vi "Velocity Profile.vi"(0 "Set Point":dbl(slide)=1510.204081632653 scale=-2000.0..2000.0, 1 "Iteration":i32, 2 "Reset":bool, 3 "Reset 2":bool, 5 "Position Sense":dbl(slide) scale=-2000.0..2000.0, 7 "Rate Sense":dbl(slide) scale=-1000.0..1000.0, 11 "Velocity Profile":dbl[][](array[numeric])=[[50.0, 75.0, 0.05], [100.0, 150.0, 0.1], [250.0, 400.0, 0.2], [500.0, inf, 0.2]], 12 "queue":refnum<queue>, 13 "Hold":bool, 14 "array":dbl[](array[numeric])) -> (4 "Motor":dbl, 8 "arrived":bool, 15 "gear":i32)   [LabVIEW 2012]
panel:
  out "Rate Obj":dbl(graph)
  out "Accel":dbl
  out "Rate":dbl
  out "Waveform Chart":dbl(graph)
  # "Range"
  # "Rate"
  # "Accel"
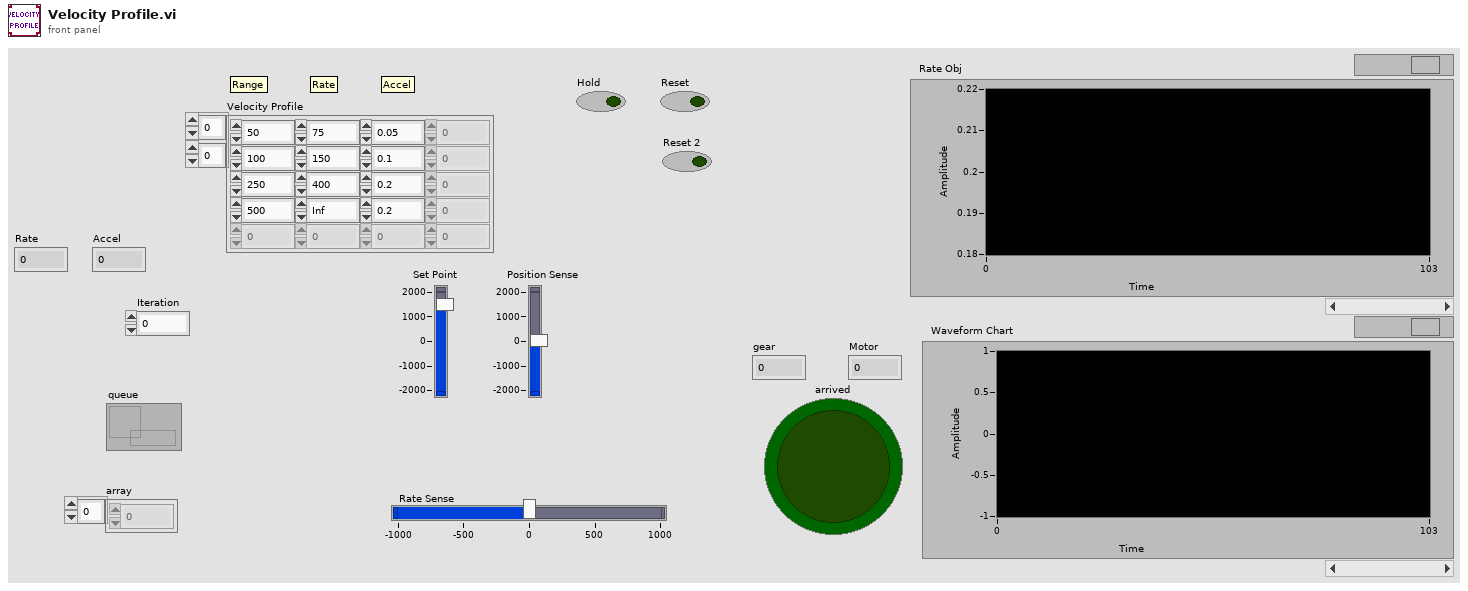
[diagram p1: front panel]
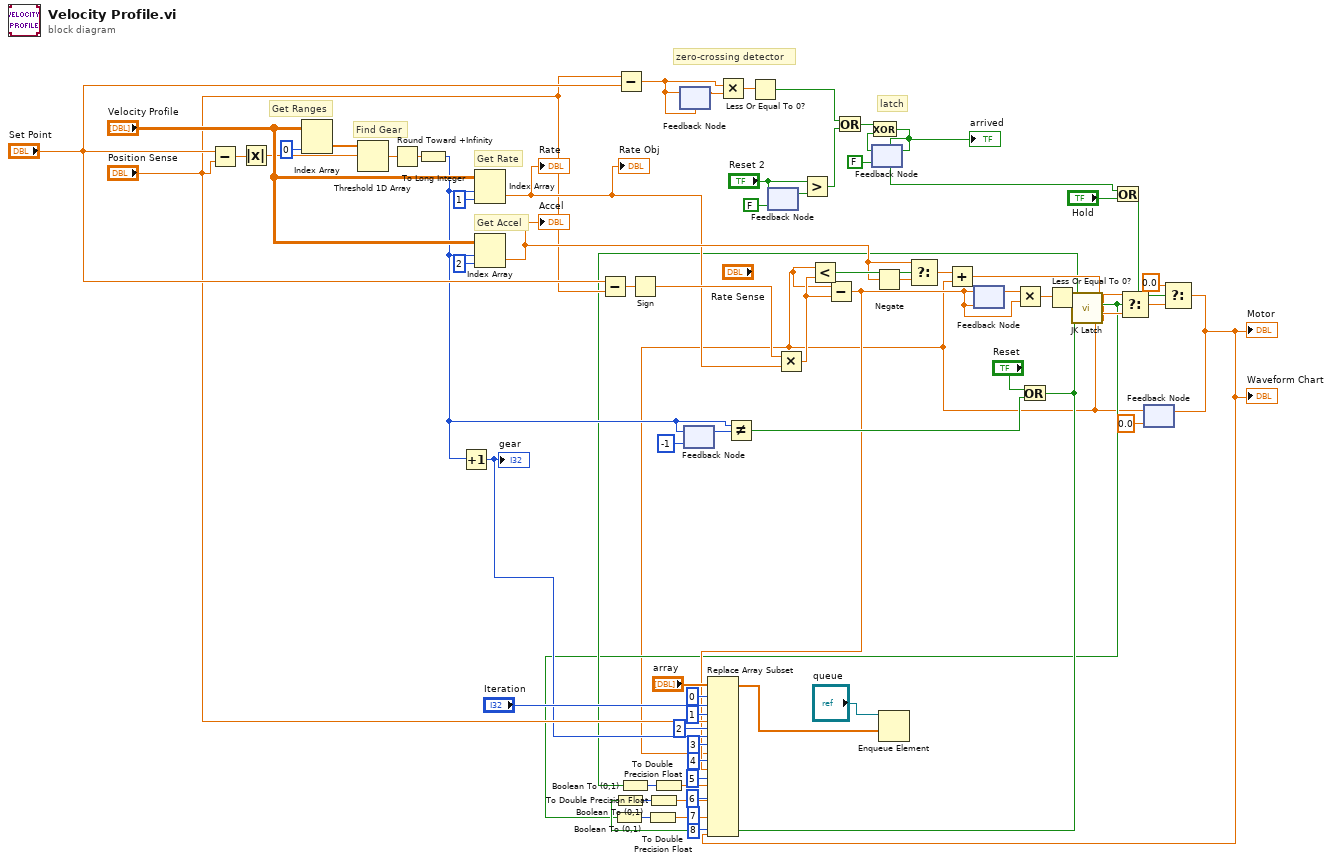
[diagram p0: block diagram]
diagram:
  (unwired) 7 ("index")
  # "latch"
  # "Get Accel"
  # "Get Rate"
  # "Find Gear"
  # "Get Ranges"
  # "zero-crossing detector"
  n1 = Subtract(x="Set Point", y="Position Sense") -> (x-y=w42:dbl)
  n2 = Absolute Value(x=w42) -> (abs(x)=w41:dbl)
  n3 = Index Array(array="Velocity Profile", index (col)=0 ("disabled index (col)")) -> (element=w49:dbl[])  [unwired: 1 in]
  n4 = Threshold 1D Array(2:w41, 3:w49) -> (0:w50:dbl)  [unwired: 1 in]
  n5 = Round Toward +Infinity(x=w50) -> (ceil(x): smallest int >= x=w40:dbl)
  n6 = To Long Integer(number=w40) -> (32bit integer=w39:i32)
  n7 = Increment(x=w39) -> (x+1=w16:i32)
  "gear" <- w16
  n8 = Index Array(array="Velocity Profile", index (row)=w39, index (col)=1 ("disabled index (col)")) -> (element=w36:dbl)
  "Rate" <- w36
  "Rate Obj" <- w36
  n9 = Index Array(array="Velocity Profile", index (row)=w39, index (col)=2 ("disabled index (col)")) -> (element=w45:dbl)
  "Accel" <- w45
  n10 = Subtract(x="Set Point", y="Position Sense") -> (x-y=w67:dbl)
  n11 = Subtract(x="Position Sense", y="Set Point") -> (x-y=w56:dbl)
  n12 = Sign(1:w67) -> (0:w58:dbl)
  n13 = feedback #1(w56) -> (w69:dbl)
  n14 = feedback-in #1(w56) -> ()
  n15 = feedback #2(-1) -> (w53:i32)
  n16 = feedback-in #2(w39) -> ()
  n17 = Multiply(x=w56, y=w69) -> (x*y=w68:dbl)
  n18 = Not Equal?(x=w39, y=w53) -> (x != y?=w52:bool)
  n19 = Less Or Equal To 0?(x=w68) -> (x <= 0?=w5:bool)
  n20 = feedback-in #3("Reset 2") -> ()
  n21 = feedback #3(FALSE ("Reset 2")) -> (w3:bool)
  n22 = Multiply(x=w58, y=w36) -> (x*y=w57:dbl)
  n23 = Greater?(x="Reset 2", y=w3) -> (0:w1:bool)
  n24 = Or(x=w5, y=w1) -> (x .or. y?=w6:bool)
  n25 = feedback #4(FALSE) -> (w9:bool)
  n26 = Exclusive Or(1:w9, 2:w6) -> (0:w7:bool)
  "arrived" <- w7
  n27 = feedback-in #4(w7) -> ()
  n28 = Negate(x=w45) -> (-x=w62:dbl)
  n29 = Or(x="Reset", y=w52) -> (x .or. y?=w13:bool)
  n30 = Boolean To (0,1)(Boolean=w13) -> (0, 1=w24:i16)
  n31 = To Double Precision Float(number=w24) -> (double precision float=w23:dbl)
  n32 = Or(x=w7, y="Hold") -> (x .or. y?=w38:bool)
  n33 = feedback #5(0.0) -> (w10:dbl)
  n34 = Less?(x=w10, y=w57) -> (x < y?=w61:bool)
  n35 = Subtract(x=w10, y=w57) -> (x-y=w15:dbl)
  n36 = Select(t=w45, s=w61, f=w62) -> (s? t:f=w63:dbl)
  n37 = Add(x=w63, y=w10) -> (x+y=w55:dbl)
  n38 = feedback #6(w15) -> (w59:dbl)
  n39 = feedback-in #6(w15) -> ()
  n40 = Multiply(x=w59, y=w15) -> (x*y=w60:dbl)
  n41 = Less Or Equal To 0?(x=w60) -> (x <= 0?=w14:bool)
  n42 = Boolean To (0,1)(Boolean=w14) -> (0, 1=w28:i16)
  n43 = To Double Precision Float(number=w28) -> (double precision float=w27:dbl)
  n44 = call "JK Latch.vi"("Reset"=w13, "Set"=w14) -> ("Q"=w12:bool)  [unwired: 5 in]
  n45 = Boolean To (0,1)(Boolean=w12) -> (0, 1=w35:i16)
  n46 = To Double Precision Float(number=w35) -> (double precision float=w22:dbl)
  n47 = Select(t=w10, s=w12, f=w55) -> (s? t:f=w65:dbl)
  n48 = Select(t=0.0, s=w38, f=w65) -> (s? t:f=w11:dbl)
  "Motor" <- w11
  "Waveform Chart" <- w11
  n49 = Replace Array Subset(array="array", new element #1="Iteration", index #1=0 ("index"), new element #2="Position Sense", index #2=1 ("index"), new element #3=w16, index #3=2 ("index"), new element #4=w10, index #4=3 ("index"), new element #5=w15, index #5=4 ("index"), new element #6=w27, index #6=5 ("index"), new element #7=w23, index #7=6 ("index"), new element #8=w22, new element #9=w11, index #9=8 ("index")) -> (w34:dbl[])  [unwired: 1 in]
  n50 = Enqueue Element(queue="queue", element=w34) -> ()  [unwired: 2 in, 3 out]
  n51 = feedback-in #5(w11) -> ()
